vi "GlobalGetPolarisatorParameters.vi"() -> ()   [LabVIEW 2011]
panel:
  in  "Phase  Compensation":dbl
  in  "Polarisatior":enum16{"Radial", "Azimuthal"}(ring)
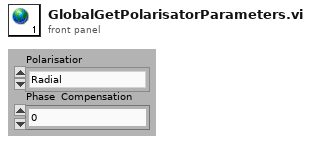
[diagram p1: front panel]
diagram:
